vi "safeties.vi"(10 "Prev Iteration Data":T4) -> (0 "Safety Data and Log":T4, 1 "Gyro Failure":bool, 2 "No Gyro Rate Read":bool, 3 "Drive":T3, 5 "Container Arm":T2, 7 "Lift Belts":T1)   [LabVIEW 2014]
uses:
  <vilib>/Rock Robotics/Network Tables/NT Read Boolean Array.vi
panel:
  out "Safety Data":bool[](array[boolean])
  out "Multicolumn Listbox":i32(listbox)
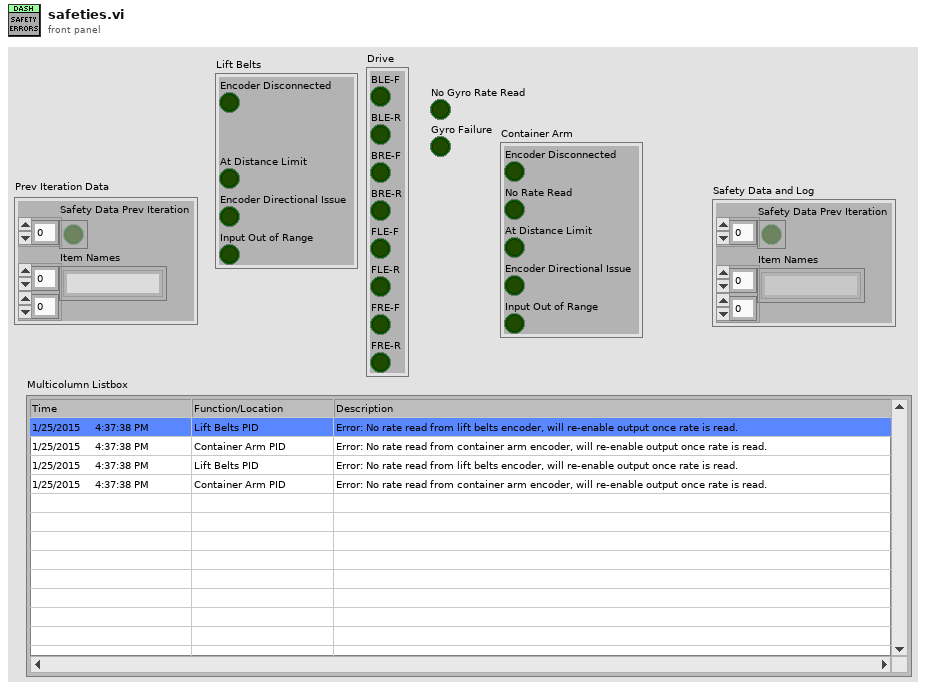
[diagram p1: front panel]
types:
  T1 = cluster{"Encoder Disconnected":bool, "At Distance Limit":bool, "Encoder Directional Issue":bool, "Input Out of Range":bool}
  T2 = cluster{"Encoder Disconnected":bool, "No Rate Read":bool, "At Distance Limit":bool, "Encoder Directional Issue":bool, "Input Out of Range":bool}
  T3 = cluster{"BLE-F":bool, "BLE-R":bool, "BRE-F":bool, "BRE-R":bool, "FLE-F":bool, "FLE-R":bool, "FRE-F":bool, "FRE-R":bool}
  T4 = cluster{"Safety Data Prev Iteration":bool[], "Item Names":string[][]}
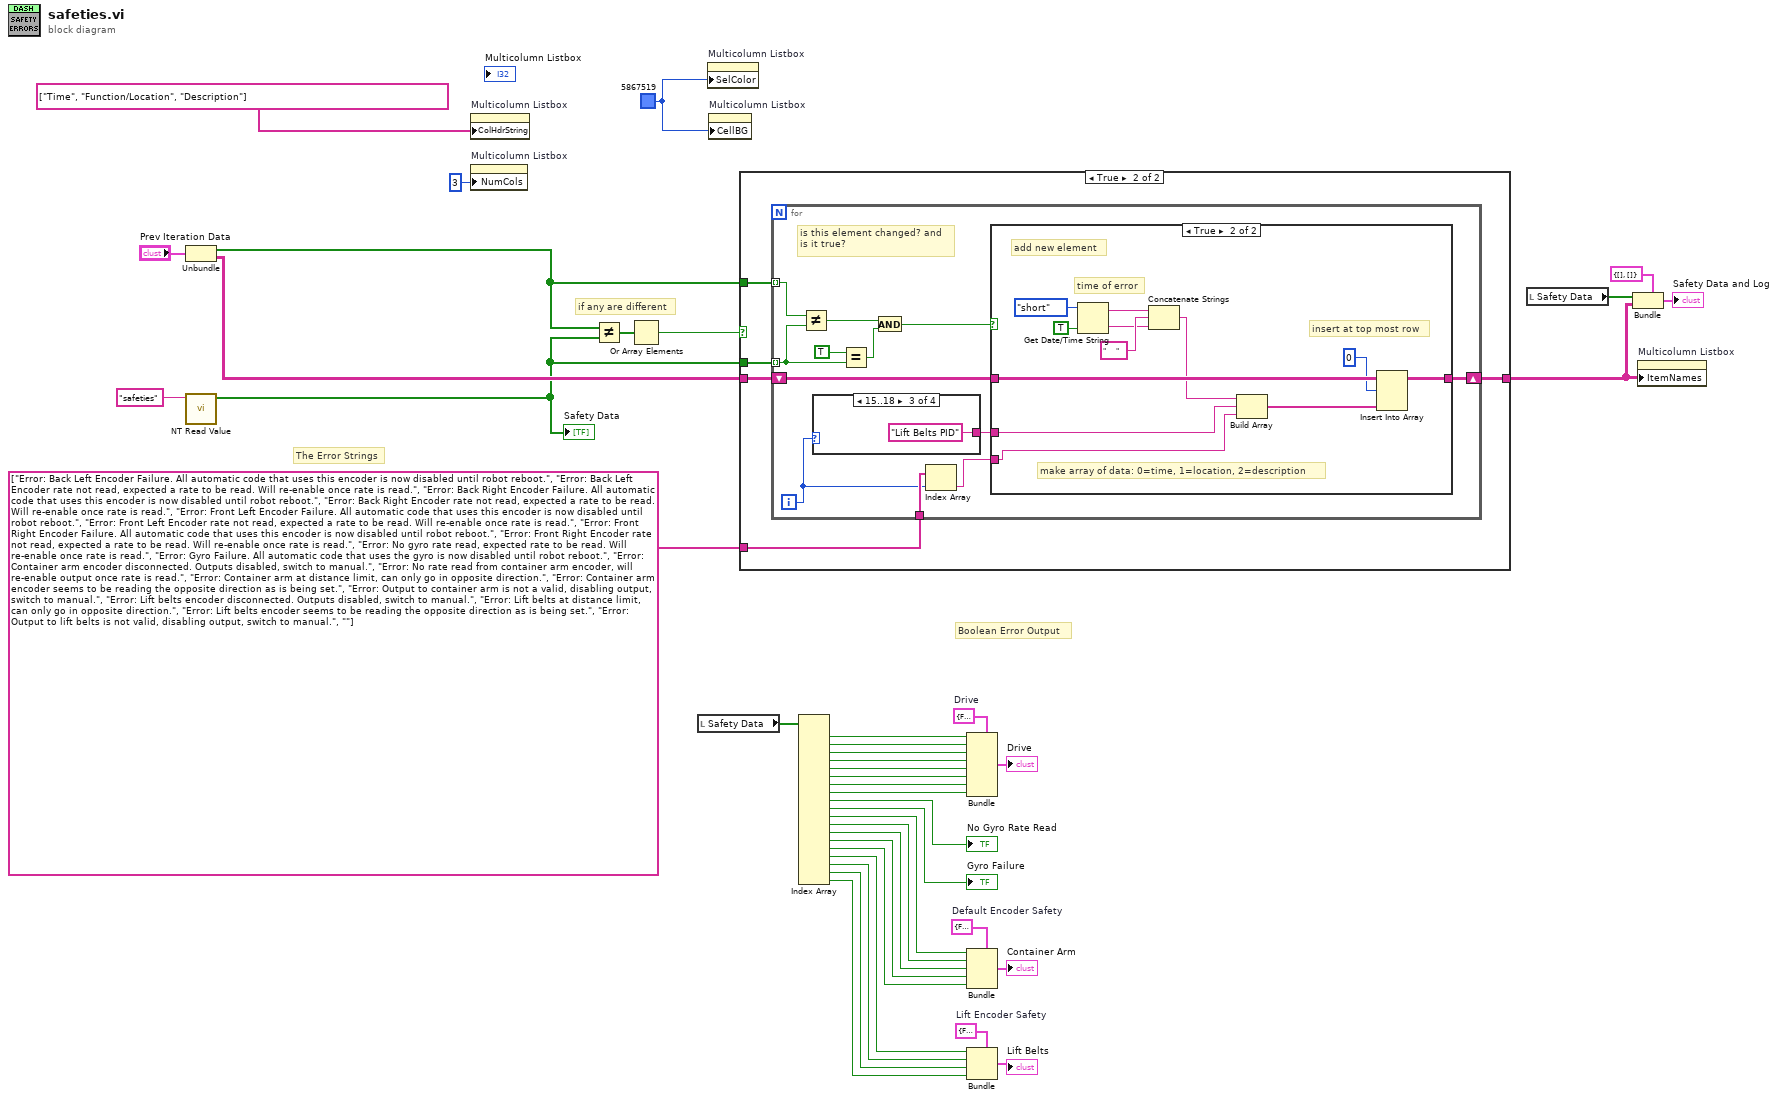
[diagram p0: block diagram]
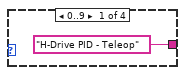
[diagram p3: hidden frame]
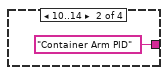
[diagram p4: hidden frame]
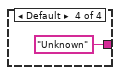
[diagram p5: hidden frame]
diagram:
  w7 = T1 {"Encoder Disconnected"=FALSE, "At Distance Limit"=FALSE, "Encoder Directional Issue"=FALSE, "Input Out of Range"=FALSE}  # Lift Encoder Safety
  w13 = T2 {"Encoder Disconnected"=FALSE, "No Rate Read"=FALSE, "At Distance Limit"=FALSE, "Encoder Directional Issue"=FALSE, "Input Out of Range"=FALSE}  # Default Encoder Safety
  w26 = T3 {"BLE-F"=FALSE, "BLE-R"=FALSE, "BRE-F"=FALSE, "BRE-R"=FALSE, "FLE-F"=FALSE, "FLE-R"=FALSE, "FRE-F"=FALSE, "FRE-R"=FALSE}  # Drive
  w28 = u32 5867519 ("Round Color Box")
  # "Boolean Error Output"
  # "The Error Strings"
  # "if any are different"
  n1 = Unbundle("Prev Iteration Data") -> ("Safety Data Prev Iteration"=w35:bool[], "Item Names"=w34:string[][])
  n2 = call-poly <vilib>:"NT Read Value.vi"("Name"="safeties") -> ("Boolean Array"=w14:bool[])  [unwired: 9 in, 1 out]
  "Safety Data" <- w14
  n3 = property on="Multicolumn Listbox" class="MCListbox (strict)"("ColHdrString"=string[] ["Time", "Function/Location", "Description"] ("Column Header Strings[]")) -> ()  [unwired: 2 in, 2 out]
  n4 = property on="Multicolumn Listbox" class="MCListbox (strict)"("NumCols"=u32 3 ("Number of Columns")) -> ()  [unwired: 2 in, 2 out]
  n5 = Not Equal?(x=w35, y=w14) -> (x != y?=w37:bool[])
  n6 = Or Array Elements(Boolean array=w37) -> (logical OR=w36:bool)
  n7 = local read "Safety Data"() -> (w27:bool[])
  n8 = property on="Multicolumn Listbox" class="MCListbox (strict)"("SelColor"=w28) -> ()  [unwired: 2 in, 2 out]
  n9 = property on="Multicolumn Listbox" class="MCListbox (strict)"("CellBG"=w28) -> ()  [unwired: 2 in, 2 out]
  n10 = case shown="True" w36 {
    tunnel: w14 -> [_ w47]
    tunnel: w35 -> [_ w46]
    tunnel: w34 -> [w42 w45]
    tunnel: [w42 w44] -> w30
    tunnel: string[] ["Error: Back Left Encoder Failure. All automatic code that uses this encoder is now disabled until robot reboot.", "Error: Back Left Encoder rate not read, expected a rate to be read. Will re-enable once rate is read.", "Error: Back Right Encoder Failure. All automatic code that uses this encoder is now disabled until robot reboot.", "Error: Back Right Encoder rate not read, expected a rate to be read. Will re-enable once rate is read.", "Error: Front Left Encoder Failure. All automatic code that uses this encoder is now disabled until robot reboot.", "Error: Front Left Encoder rate not read, expected a rate to be read. Will re-enable once rate is read.", "Error: Front Right Encoder Failure. All automatic code that uses this encoder is now disabled until robot reboot.", "Error: Front Right Encoder rate not read, expected a rate to be read. Will re-enable once rate is read.", "Error: No gyro rate read, expected rate to be read. Will re-enable once rate is read.", "Error: Gyro Failure. All automatic code that uses the gyro is now disabled until robot reboot.", "Error: Container arm encoder disconnected. Outputs disabled, switch to manual.", "Error: No rate read from container arm encoder, will re-enable output once rate is read.", "Error: Container arm at distance limit, can only go in opposite direction.", "Error: Container arm encoder seems to be reading the opposite direction as is being set.", "Error: Output to container arm is not a valid, disabling output, switch to manual.", "Error: Lift belts encoder disconnected. Outputs disabled, switch to manual.", "Error: Lift belts at distance limit, can only go in opposite direction.", "Error: Lift belts encoder seems to be reading the opposite direction as is being set.", "Error: Output to lift belts is not valid, disabling output, switch to manual.", ""] -> [_ w43]
    frame False {
    }
    frame True {
      n11 = for {
        tunnel: w47 -> [w49] mode=indexing
        tunnel: w46 -> [w59] mode=indexing
        shift-right: [w56] -> w44
        shift-left: w45 -> [w58]
        tunnel: w43 -> [w54]
        i -> [w53]
        # "is this element changed? and\nis it true?"
        n12 = Not Equal?(x=w59, y=w49) -> (x != y?=w57:bool)
        n13 = case shown="15..18" w53 {
          tunnel: ["H-Drive PID - Teleop" "Container Arm PID" "Lift Belts PID" "Unknown"] -> w55
          frame 0..9 {
          }
          frame 10..14 {
          }
          frame 15..18 {
          }
          frame Default {
          }
        }
        n14 = Equal?(x=TRUE, y=w49) -> (x = y?=w50:bool)
        n15 = And(x=w57, y=w50) -> (x .and. y?=w51:bool)
        n16 = Index Array(array=w54, index=w53) -> (element=w52:string)
        n17 = case shown="True" w51 {
          tunnel: w58 -> [w64 w76]
          tunnel: [w64 w75] -> w56
          tunnel: w55 -> [_ w65]
          tunnel: w52 -> [_ w69]
          frame False {
          }
          frame True {
            # "make array of data: 0=time, 1=location, 2=description"
            # "insert at top most row"
            # "time of error"
            # "add new element"
            n18 = Get Date/Time String(date format (0)=enum16{"short", "long", "abbreviated"}."short", want seconds? (F)=TRUE) -> (date string=w71:string, time string=w70:string)  [unwired: 1 in]
            n19 = Concatenate Strings(w71, "     " ("string"), w70) -> (w66:string)
            n20 = Build Array(w66, w65, w69) -> (w67:string[])
            n21 = Insert Into Array(array=w76, index (row)=0, new element=w67) -> (w75:string[][])  [unwired: 1 in]
          }
        }
      }
    }
  }
  n22 = Index Array(array=w27) -> (element #1=w25:bool, element #2=w24:bool, element #3=w23:bool, element #4=w22:bool, element #5=w21:bool, element #6=w20:bool, element #7=w19:bool, element #8=w18:bool, element #9=→"No Gyro Rate Read":bool, element #10=→"Gyro Failure":bool, element #11=w12:bool, element #12=w11:bool, element #13=w10:bool, element #14=w9:bool, element #15=w8:bool, element #16=w6:bool, element #17=w3:bool, element #18=w2:bool, element #19=w1:bool)  [unwired: 19 in]
  n23 = Bundle(cluster=w26, "BLE-F"=w25, "BLE-R"=w24, "BRE-F"=w23, "BRE-R"=w22, "FLE-F"=w21, "FLE-R"=w20, "FRE-F"=w19, "FRE-R"=w18) -> (→"Drive":T3)
  n24 = Bundle(cluster=w13, "Encoder Disconnected"=w12, "No Rate Read"=w11, "At Distance Limit"=w10, "Encoder Directional Issue"=w9, "Input Out of Range"=w8) -> (→"Container Arm":T2)
  n25 = Bundle(cluster=w7, "Encoder Disconnected"=w6, "At Distance Limit"=w3, "Encoder Directional Issue"=w2, "Input Out of Range"=w1) -> (→"Lift Belts":T1)
  n26 = local read "Safety Data"() -> (w31:bool[])
  n27 = Bundle(cluster=T4 {"Safety Data Prev Iteration"=[], "Item Names"=[]} ("Prev Iteration Data"), "Safety Data Prev Iteration"=w31, "Item Names"=w30) -> (→"Safety Data and Log":T4)
  n28 = property on="Multicolumn Listbox" class="MCListbox (strict)"("ItemNames"=w30) -> ()  [unwired: 2 in, 2 out]
